vi "Check-ready.vi"(8 "error in (no error)":errorcluster, 11 "Motor-DAQmx in":refnum<class "Motor-DAQmx.lvclass">) -> (0 "error out":errorcluster, 2 "Ready":bool, 3 "Motor-DAQmx out":refnum<class "Motor-DAQmx.lvclass">)   [LabVIEW 2013, in "PowderDeposition.lvlib" / "Motor-DAQmx.lvclass"]
uses:
  Motor-DAQmx.lvclass
  Motor-DAQmx.lvclass/Motor-DAQmx.ctl
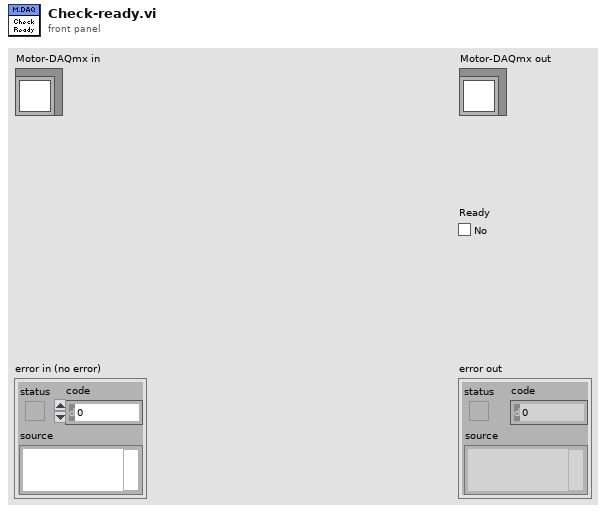
[diagram p1: front panel]
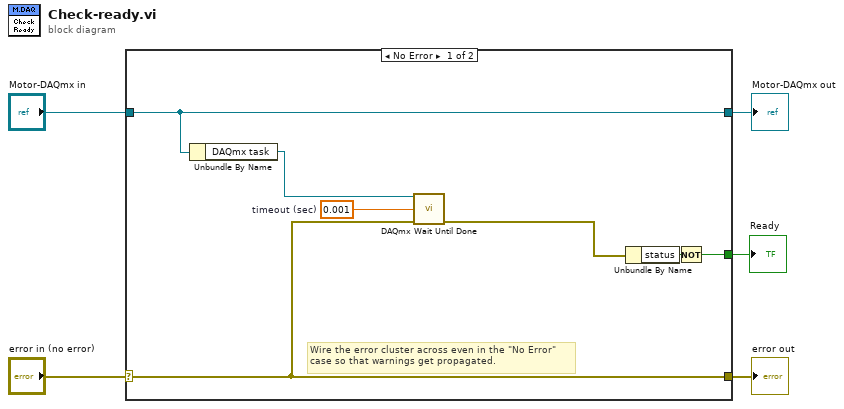
[diagram p0: block diagram]
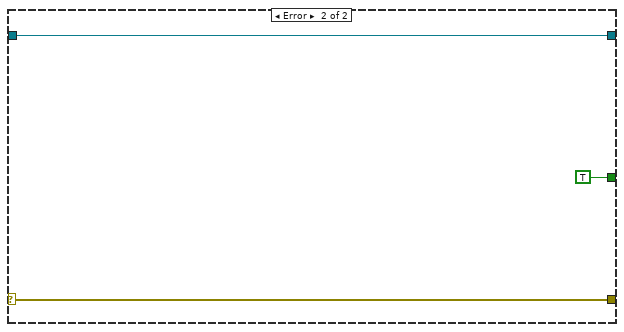
[diagram p2: hidden frame]
diagram:
  n1 = case shown="No Error" "error in (no error)" {
    selector: "error in (no error)" -> [w8 w15]
    tunnel: [w8 w15] -> w4
    tunnel: [w12 w14] -> w2
    tunnel: "Motor-DAQmx in" -> [w12 w14]
    tunnel: [w6 TRUE] -> w1
    frame No Error {
      w10 = 0.001  # timeout (sec)
      # "Wire the error cluster across even in the \"No Error\"\ncase so that warnings get propagated."
      n2 = Unbundle By Name(w12) -> ("DAQmx task"=w11:refnum<k21>)
      n3 = call <vilib>:"DAQmx Wait Until Done.vi"("task/channels in"=w11, "timeout (sec)"=w10, "error in"=w8) -> ("error out"=w9:errorcluster)  [unwired: 11 in, 1 out]
      n4 = Unbundle By Name(w9) -> ("status"=w7:bool)
      n5 = Not(x=w7) -> (.not. x?=w6:bool)
    }
    frame Error {
    }
  }
  "error out" <- w4
  "Motor-DAQmx out" <- w2
  "Ready" <- w1
